vi "Test MultiValue INSERT format.vi"() -> ()   [LabVIEW 2019]
uses:
  src/LV-Data.PG/LV-Data.PGSQL.lvclass
panel:
  in  "String":string="llab_025:v001(Montana Cryostation--User())\nllab_025:d008(Montana Cryostation--Cold Head Speed(Hz))\nllab_061:d000(AML Gauges (Analysis)--IG Pressure(mbar))"
  in  "Timestamps":timestamp[](array[timestamp])=[timestamp(3753094947.978874 s since 1904-01-01), timestamp(3753094950.8230257 s since 1904-01-01), timestamp(3810819142.718672 s since 1904-01-01)]
  in  "Data (multi multirow)":T1(array[cluster])=[{"String"="string 1", "Numeric"=1.0, "Numeric 2"=2.0}, {"String"="string 2", "Numeric"=3.0, "Numeric 2"=4.0}, {"String"="string 3", "Numeric"=5.0, "Numeric 2"=6.0}]
  in  "path(s)":string[](array[string])=["llab_025:v001(Montana Cryostation--User())", "llab_025:d008(Montana Cryostation--Cold Head Speed(Hz))", "llab_061:d000(AML Gauges (Analysis)--IG Pressure(mbar))"]
  out "Formatted Inserts":string="INSERT INTO\n  llab_025 (d008,time,v001)\nVALUES\n  (1,'2024-10-03 15:14:49.942207'::timestamptz,$$string 1$$)\r\n;\nINSERT INTO\n  llab_061 (d000,time)\nVALUES\n  (2,'2024-10-03T19:14:49.950Z'::timestamptz)\r\n;\nINSERT INTO\n  llab_025 (d008,time,v001)\nVALUES\n  (1,'2022-12-05 09:22:27.978874'::timestamptz,$$string 1$$)\r\n;\nINSERT INTO\n  llab_061 (d000,time)\nVALUES\n  (2,'2022-12-05T14:22:27.978Z'::timestamptz)\r\n;\nINSERT INTO\n  llab_025 (d008,time,v001)\nVALUES\n  (1,'2022-12-05 09:22:27.978874'::timestamptz,$$string 1$$)\r\n;\nINSERT INTO\n  llab_061 (d000,time)\nVALUES\n  (2,'2022-12-05T14:22:27.978Z'::timestamptz)\r\n;\nINSERT INTO\n  llab_025 (d008,time,v001)\nVALUES\n  (1,'2022-12-05 09:22:27.978874'::timestamptz,$$string 1$$),\n  (3,'2022-12-05 09:22:30.823025'::timestamptz,$$string 2$$),\n  (5,'2024-10-03 12:52:22.718671'::timestamptz,$$string 3$$)\r\n;\nINSERT INTO\n  llab_061 (d000,time)\nVALUES\n  (2,'2022-12-05T14:22:27.978Z'::timestamptz),\n  (4,'2022-12-05T14:22:30.823Z'::timestamptz),\n  (6,'2024-10-03T16:52:22.718Z'::timestamptz)\r\n;"
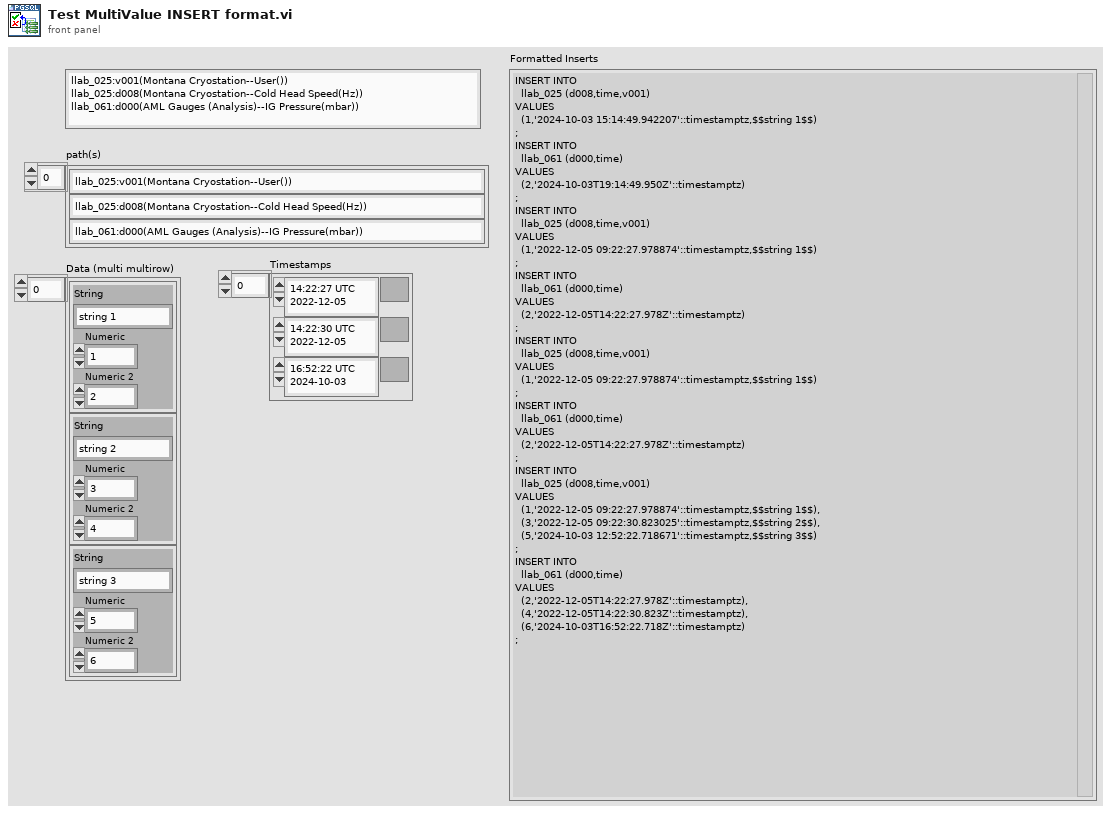
[diagram p1: front panel]
types:
  T1 = cluster{"String":string, "Numeric":dbl, "Numeric 2":dbl}[]
  T2 = cluster{"String":string, "Numeric":dbl, "Numeric 2":dbl}
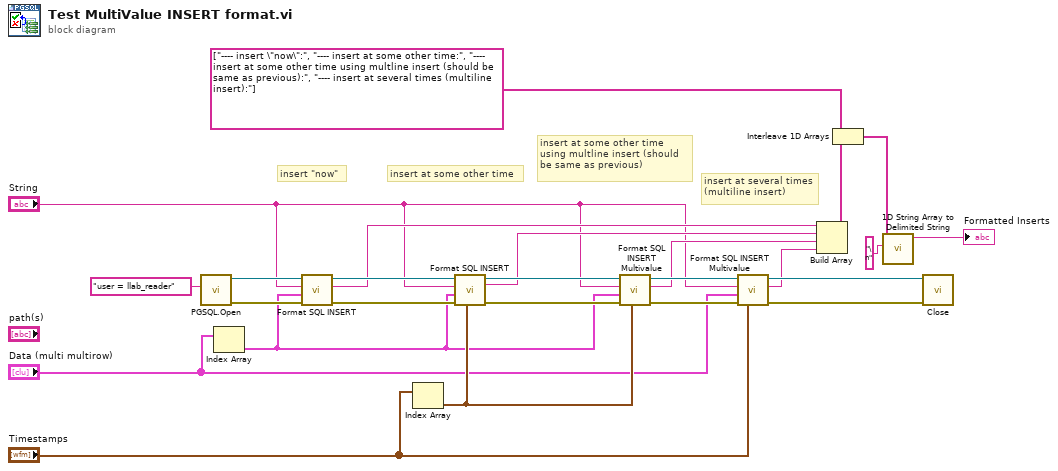
[diagram p0: block diagram]
diagram:
  # "insert at several times\n(multiline insert)"
  # "insert at some other time\nusing multline insert (should\nbe same as previous)"
  # "insert at some other time"
  # "insert \"now\""
  n1 = call "PGSQL.Open.vi"("Connection String"="user = llab_reader") -> ("error out"=w8:errorcluster, "Data.PG out"=w10:refnum<class "LV-Data.PGSQL.lvclass">)  [unwired: 9 in]
  n2 = Index Array(array="Data (multi multirow)") -> (element=w6:T2)  [unwired: 1 in]
  n3 = call "Format SQL INSERT.vi"("error in"=w8, "Data"=w6, "Path(s)"="String", "LV-Data.PGSQL in"=w10) -> ("error out"=w7:errorcluster, "Formatted Insert"=w5:string, "LV-Data.PGSQL out"=w9:refnum<class "LV-Data.PGSQL.lvclass">)  [unwired: 4 in, 1 out]
  n4 = Index Array(array="Timestamps") -> (element=w18:timestamp)  [unwired: 1 in]
  n5 = call "Format SQL INSERT.vi"("Time Stamp"=w18, "error in"=w7, "Data"=w6, "Path(s)"="String", "LV-Data.PGSQL in"=w9) -> ("error out"=w19:errorcluster, "Formatted Insert"=w15:string, "LV-Data.PGSQL out"=w24:refnum<class "LV-Data.PGSQL.lvclass">)  [unwired: 3 in, 1 out]
  n6 = call "Format SQL INSERT Multivalue.vi"("Times"=w18, "error in"=w19, "Data"=w6, "Path(s)"="String", "Data.PG in"=w24) -> ("error out"=w20:errorcluster, "SQL"=w16:string, "Data.PG out"=w23:refnum<class "LV-Data.PGSQL.lvclass">)  [unwired: 3 in, 1 out]
  n7 = call "Format SQL INSERT Multivalue.vi"("Times"="Timestamps", "error in"=w20, "Data"="Data (multi multirow)", "Path(s)"="String", "Data.PG in"=w23) -> ("error out"=w21:errorcluster, "SQL"=w17:string, "Data.PG out"=w22:refnum<class "LV-Data.PGSQL.lvclass">)  [unwired: 3 in, 1 out]
  n8 = Build Array(w5, w15, w16, w17) -> (w2:string[])
  n9 = Interleave 1D Arrays(string[] ["---- insert \"now\":", "---- insert at some other time:", "---- insert at some other time using multline insert (should be same as previous):", "---- insert at several times (multiline insert):"], w2) -> (w1:string[])
  n10 = call <vilib>:"1D String Array to Delimited String.vi"("delimiter"="\n", "string array"=w1) -> ("delimited string"=→"Formatted Inserts":string)  [unwired: 9 in]
  n11 = call-dynamic "Close.vi"("error in (no error)"=w21, "Data.PG in"=w22) -> ()  [unwired: 8 in, 2 out]
